vi "Test_AddGetTopic_RetrievalOK.vi"(8 "error in (no error)":errorcluster, 11 "TestCase in":refnum<class "TestTopicLookupTable.lvclass">) -> (0 "error out":errorcluster, 3 "TestCase out":refnum<class "TestTopicLookupTable.lvclass">)   [LabVIEW 2015, in "Mediator.lvlib" / "TestTopicLookupTable.lvclass"]
uses:
  TestTopicLookupTable.lvclass
  <vilib>/ActorFramework/Message Queue/Message Queue.lvclass/Message Queue.ctl
  <vilib>/addons/_JKI Toolkits/VI Tester/TestCase.llb/TestCase.lvclass
  TopicLookupTable/TopicLookupTable.lvclass
  Topic/Topic.lvclass
  <vilib>/ActorFramework/Message Queue/Message Queue.lvclass
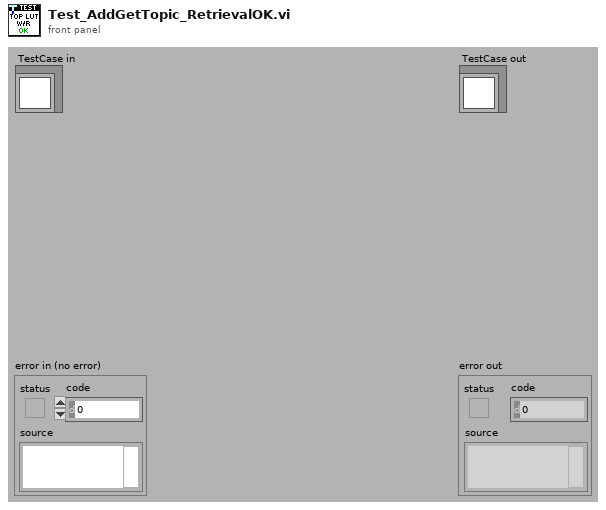
[diagram p1: front panel]
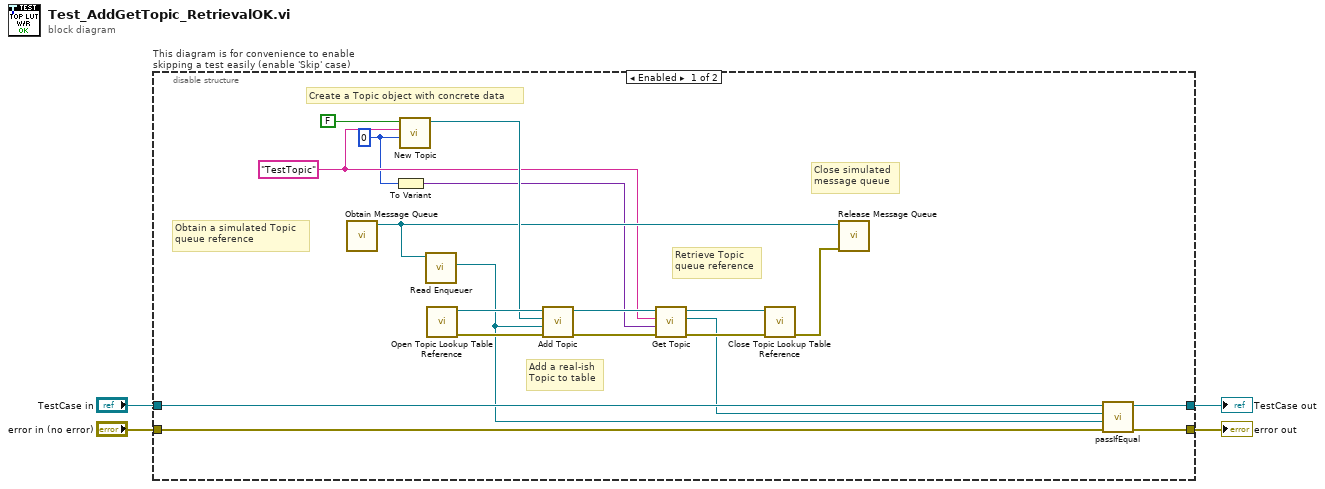
[diagram p0: block diagram]
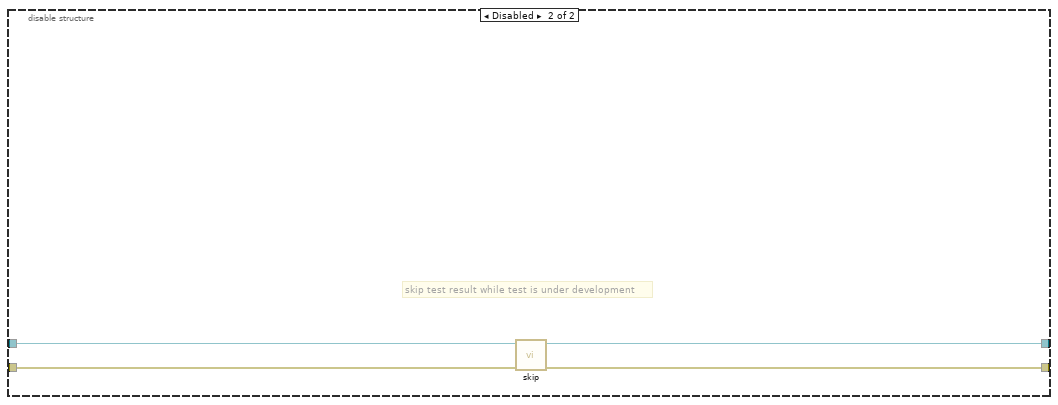
[diagram p2: hidden frame]
diagram:
  n1 = disable-structure "This diagram is for convenience to enable skipping a test easily (enable 'Skip' case)" shown="Enabled" {
    disable-tunnel: "TestCase in" -> [w23 w27]
    disable-tunnel: [w22 w25] -> w1
    disable-tunnel: [w21 w26] -> w3
    disable-tunnel: "error in (no error)" -> [w20 w24]
    frame Enabled {
      w8 = 0
      w9 = "TestTopic" ("Name")
      # "Create a Topic object with concrete data"
      # "Add a real-ish\nTopic to table"
      # "Close simulated\nmessage queue"
      # "Retrieve Topic\nqueue reference"
      # "Obtain a simulated Topic\nqueue reference"
      n2 = call <vilib>:"Obtain Message Queue.vi"() -> ("Message Queue"=w10:refnum<class "Message Queue.lvclass">)  [unwired: 10 in, 1 out]
      n3 = To Variant(anything=w8) -> (Variant=w7:variant)
      n4 = call "New Topic.vi"("New Topic Data"=w8, "Name"=w9, "Use Type Input As Initial Value?"=FALSE) -> ("Topic out"=w13:refnum<class "Topic.lvclass">)  [unwired: 7 in, 1 out]
      n5 = call <vilib>:"Read Enqueuer.vi"("Message Queue"=w10) -> ("Message Enqueuer"=w12:refnum<class "Message Enqueuer.lvclass">)  [unwired: 10 in]
      n6 = call "Open Topic Lookup Table Reference.vi"() -> ("error out"=w18:errorcluster, "TopicLookupTable Reference"=w19:refnum<data-value>)  [unwired: 10 in]
      n7 = call "Add Topic.vi"("error in (no error)"=w18, "Topic Enqueuer"=w12, "Topic Object"=w13, "TopicLookupTable"=w19) -> ("error out"=w16:errorcluster, "TopicLookupTable"=w17:refnum<data-value>)  [unwired: 5 in, 1 out]
      n8 = call "Get Topic.vi"("error in (no error)"=w16, "Topic Type"=w7, "Topic Name"=w9, "TopicLookupTable"=w17) -> ("error out"=w14:errorcluster, "Topic Refnum"=w6:refnum<class "Message Enqueuer.lvclass">, "TopicLookupTable"=w15:refnum<data-value>)  [unwired: 5 in]
      n9 = call "Close Topic Lookup Table Reference.vi"("error in (no error)"=w14, "TopicLookupTable"=w15) -> ("error out"=w11:errorcluster)  [unwired: 9 in]
      n10 = call <vilib>:"Release Message Queue.vi"("error in (no error)"=w11, "Message Queue"=w10) -> ()  [unwired: 8 in, 2 out]
      n11 = call-dynamic "passIfEqual.vi"("error in (no error)"=w20, "y"=w12, "x"=w6, "TestCase in"=w23) -> ("error out"=w21:errorcluster, "TestCase out"=w22:refnum<class "TestTopicLookupTable.lvclass">)  [unwired: 6 in]
    }
    frame Disabled {
      # "skip test result while test is under development"
      n12 = call <vilib>:"skip.vi"("error in (no error)"=w24, "TestCase in"=w27) -> ("error out"=w26:errorcluster, "TestCase out"=w25:refnum<class "TestTopicLookupTable.lvclass">)  [unwired: 8 in]
    }
  }
  "error out" <- w3
  "TestCase out" <- w1
